vi "STAT 2 Tractor Decode Analog Data.vi"(0 "Received(T)":bool=TRUE, 7 "Controller STAT 2":T1 {"Tension Sub 2"."sys register" format="%04x"; "Tension Sub 1"."sys register" format="%04x"; "PSU"."sys register" format="%04x"; "solonoid"."valve status" format="%02x"; "solonoid"."sys register" format="%04x"; "pressure 2"."sys register" format="%04x"; "pressure 1"."sys register" format="%04x"; "Controller local"."High G monitoring" format="%02x"; "Controller local"."NA" format="%02x"; "Controller local"."GPIO values" format="%02x"; "Controller local"."Relay status" format="%02x"; "Controller local"."sys register" format="%04x"}, 11 "error in (no error)":errorcluster) -> (6 "Tool analog value":dbl[](array[numeric]), 10 "Tool analog index":u16[](array[numeric]), 15 "error out":errorcluster)   [LabVIEW 2011]
uses:
  Stroker/Stat def/Stroker system stat2.ctl
  LEINmaster/Nodes/Controller local stat2.ctl
  LEINmaster/Nodes/pressure stat2.ctl
  LEINmaster/Nodes/solonoid stat2.ctl
  LEINmaster/Nodes/PSU stat2.ctl
  LEINmaster/Nodes/tensionsub stat2.ctl
  High Level/Variable List Tractor Analog.ctl
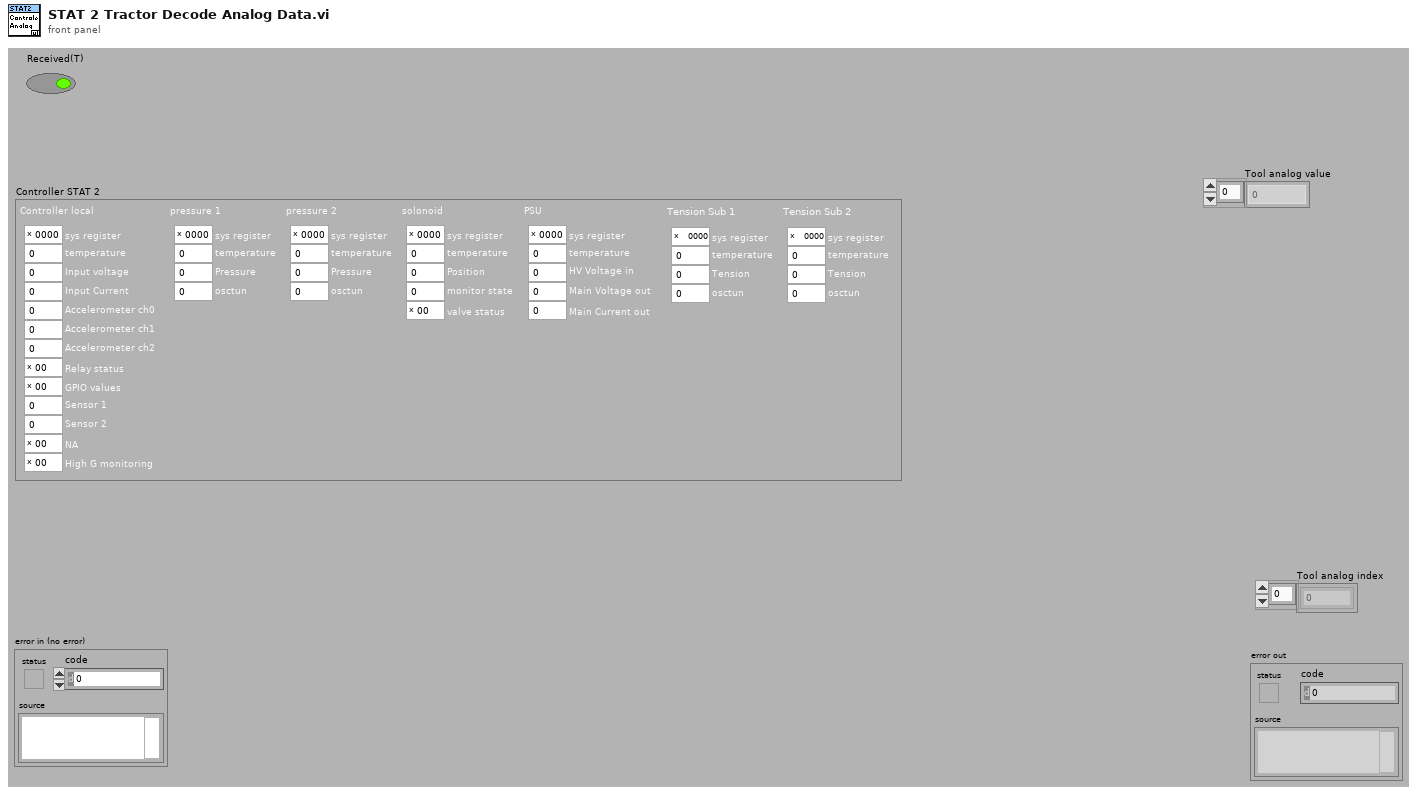
[diagram p1: front panel]
types:
  T1 = typedef "Stroker system stat2.ctl" = cluster{"Controller local":T2, "pressure 1":T3, "pressure 2":T3, "solonoid":T4, "PSU":T5, "Tension Sub 1":T6, "Tension Sub 2":T6}
  T2 = typedef "Controller local stat2.ctl" = cluster{"sys register":u16, "temperature":u16, "Input voltage":u16, "Input Current":u16, "Accelerometer ch0":u16, "Accelerometer ch1":u16, "Accelerometer ch2":u16, "Relay status":u8, "GPIO values":u8, "Sensor 1":i32, "Sensor 2":i32, "NA":u8, "High G monitoring":u8}
  T3 = typedef "pressure stat2.ctl" = cluster{"sys register":u16, "temperature":u16, "Pressure":u16, "osctun":u8}
  T4 = typedef "solonoid stat2.ctl" = cluster{"sys register":u16, "temperature":u16, "Position":i16, "monitor state":u8, "valve status":u8}
  T5 = typedef "PSU stat2.ctl" = cluster{"sys register":u16, "temperature":u16, "HV Voltage in":u16, "Main Voltage out":u16, "Main Current out":u16}
  T6 = typedef "tensionsub stat2.ctl" = cluster{"sys register":u16, "temperature":u16, "Tension":i16, "osctun":u8}
  T7 = typedef "Variable List Tractor Analog.ctl" = enum16{"Tool max Temperature", "Tool supply Voltage", "Tool (Controller) Current", "Tool Acceleration X", "Tool Acceleration Y", "Tool Acceleration Z", "Controller Temp", "Tool Acceleration Sum", "Tool Inclination", "Tool Rotation", "Tool GP Sensor 1", "Tool GP Sensor 2", "PSU Temp", "Head Voltage", "PSU Main Voltage out", "PSU Main Current out", "Upper Tension Sub Temp", "Tool Upper Tension Sub", "Lower Tension Sub Temp", "Tool Lower Tension Sub"}
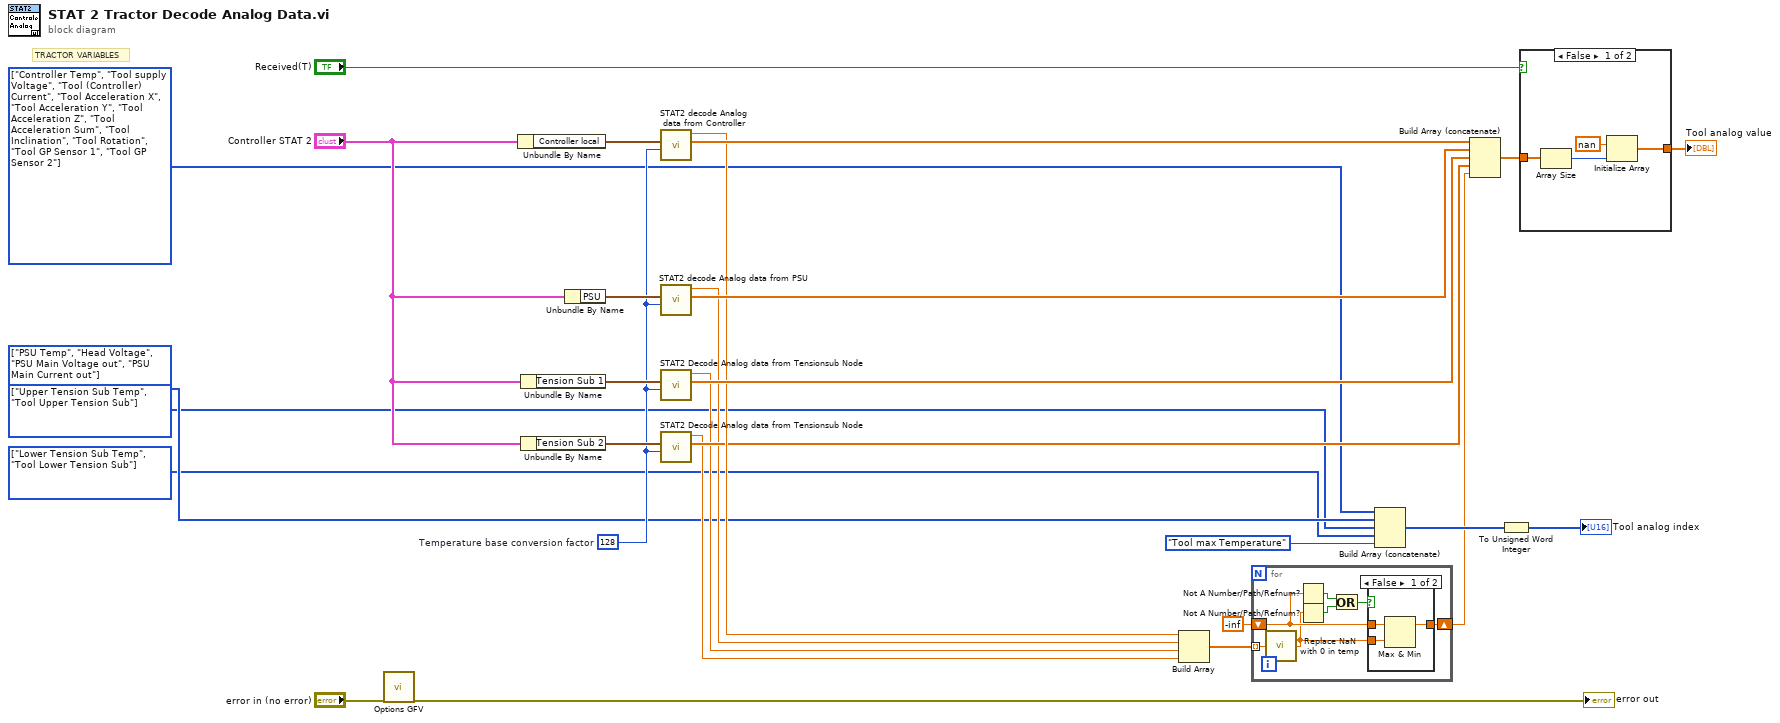
[diagram p0: block diagram]
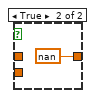
[diagram p2: hidden frame]
diagram:
  w2 = T7[] [enum."Lower Tension Sub Temp", enum."Tool Lower Tension Sub"] items=["Tool max Temperature", "Tool supply Voltage", "Tool (Controller) Current", "Tool Acceleration X", "Tool Acceleration Y", "Tool Acceleration Z", "Controller Temp", "Tool Acceleration Sum", "Tool Inclination", "Tool Rotation", "Tool GP Sensor 1", "Tool GP Sensor 2", "PSU Temp", "Head Voltage", "PSU Main Voltage out", "PSU Main Current out", "Upper Tension Sub Temp", "Tool Upper Tension Sub", "Lower Tension Sub Temp", "Tool Lower Tension Sub"]
  w3 = T7[] [enum."Upper Tension Sub Temp", enum."Tool Upper Tension Sub"] items=["Tool max Temperature", "Tool supply Voltage", "Tool (Controller) Current", "Tool Acceleration X", "Tool Acceleration Y", "Tool Acceleration Z", "Controller Temp", "Tool Acceleration Sum", "Tool Inclination", "Tool Rotation", "Tool GP Sensor 1", "Tool GP Sensor 2", "PSU Temp", "Head Voltage", "PSU Main Voltage out", "PSU Main Current out", "Upper Tension Sub Temp", "Tool Upper Tension Sub", "Lower Tension Sub Temp", "Tool Lower Tension Sub"]
  w4 = T7[] [enum."PSU Temp", enum."Head Voltage", enum."PSU Main Voltage out", enum."PSU Main Current out"] items=["Tool max Temperature", "Tool supply Voltage", "Tool (Controller) Current", "Tool Acceleration X", "Tool Acceleration Y", "Tool Acceleration Z", "Controller Temp", "Tool Acceleration Sum", "Tool Inclination", "Tool Rotation", "Tool GP Sensor 1", "Tool GP Sensor 2", "PSU Temp", "Head Voltage", "PSU Main Voltage out", "PSU Main Current out", "Upper Tension Sub Temp", "Tool Upper Tension Sub", "Lower Tension Sub Temp", "Tool Lower Tension Sub"]
  w5 = T7[] [enum."Controller Temp", enum."Tool supply Voltage", enum."Tool (Controller) Current", enum."Tool Acceleration X", enum."Tool Acceleration Y", enum."Tool Acceleration Z", enum."Tool Acceleration Sum", enum."Tool Inclination", enum."Tool Rotation", enum."Tool GP Sensor 1", enum."Tool GP Sensor 2"] items=["Tool max Temperature", "Tool supply Voltage", "Tool (Controller) Current", "Tool Acceleration X", "Tool Acceleration Y", "Tool Acceleration Z", "Controller Temp", "Tool Acceleration Sum", "Tool Inclination", "Tool Rotation", "Tool GP Sensor 1", "Tool GP Sensor 2", "PSU Temp", "Head Voltage", "PSU Main Voltage out", "PSU Main Current out", "Upper Tension Sub Temp", "Tool Upper Tension Sub", "Lower Tension Sub Temp", "Tool Lower Tension Sub"]
  w10 = u16 128  # Temperature base conversion factor
  # "TRACTOR VARIABLES"
  n1 = call "Options GFV.vi"("error in (no error)"="error in (no error)") -> ("error out"=→"error out":errorcluster)  [unwired: 16 in, 2 out]
  n2 = Unbundle By Name("Controller STAT 2") -> ("Controller local"=w15:T2)
  n3 = Unbundle By Name("Controller STAT 2") -> ("Tension Sub 1"=w12:T6)
  n4 = Unbundle By Name("Controller STAT 2") -> ("Tension Sub 2"=w11:T6)
  n5 = Unbundle By Name("Controller STAT 2") -> ("PSU"=w14:T5)
  n6 = call "STAT2 decode Analog data from Controller.vi"("Temperature base conversion factor"=w10, "Controller local"=w15) -> ("Controller analog data"=w17:dbl[], "Temperature"=w16:dbl)  [unwired: 8 in]
  n7 = call "STAT2 decode Analog data from PSU.vi"("Temperature base conversion factor"=w10, "PSU"=w14) -> ("Node Analog value"=w19:dbl[], "Temperature"=w6:dbl)  [unwired: 8 in]
  n8 = call "STAT2 Decode Analog data from Tensionsub Node.vi"("Temperature base conversion factor"=w10, "Tension Sub"=w12) -> ("Node Analog value"=w20:dbl[], "Temperature"=w7:dbl)  [unwired: 8 in]
  n9 = call "STAT2 Decode Analog data from Tensionsub Node.vi"("Temperature base conversion factor"=w10, "Tension Sub"=w11) -> ("Node Analog value"=w9:dbl[], "Temperature"=w8:dbl)  [unwired: 8 in]
  n10 = Build Array(w16, w6, w7, w8) -> (w25:dbl[])
  n11 = for {
    tunnel: w25 -> [w31] mode=indexing
    shift-right: [w36] -> w18
    shift-left: -inf -> [w35]
    n12 = call "Replace NaN with 0 in temp.vi"("Temperature in"=w31) -> ("Temperature out"=w30:dbl)  [unwired: 14 in]
    n13 = Not A Number/Path/Refnum?(number/path/refnum=w35) -> (NaN/Path/Refnum?=w33:bool)
    n14 = Not A Number/Path/Refnum?(number/path/refnum=w30) -> (NaN/Path/Refnum?=w34:bool)
    n15 = Or(x=w33, y=w34) -> (x .or. y?=w32:bool)
    n16 = case shown="False" w32 {
      tunnel: [w39 nan] -> w36
      tunnel: w35 -> [w38 _]
      tunnel: w30 -> [w37 _]
      frame False {
        n17 = Max & Min(x=w38, y=w37) -> (max(x,y)=w39:dbl)  [unwired: 1 out]
      }
      frame True {
      }
    }
  }
  n18 = Build Array (concatenate)(w5, w4, w3, w2, Variable_List_Tractor_Analog."Tool max Temperature" ("Action")) -> (w29:T7[])
  n19 = Build Array (concatenate)(w17, w19, w20, w9, w18) -> (w26:dbl[])
  n20 = To Unsigned Word Integer(number=w29) -> (unsigned 16bit integer=→"Tool analog index":u16[])
  n21 = case shown="False" "Received(T)" {
    tunnel: [w41 w45] -> w27
    tunnel: w26 -> [w44 w45]
    frame False {
      n22 = Array Size(array=w44) -> (size(s)=w43:i32)
      n23 = Initialize Array(nan ("element"), w43) -> (w41:dbl[])
    }
    frame True {
    }
  }
  "Tool analog value" <- w27
